vi "Read PSLabView Instance.vi"(8 "error in (no error)":errorcluster, 11 "PalmSens in":refnum<class "PalmSens.lvclass">) -> (0 "error out":errorcluster, 2 "PSLabView Instance":refnum<k24>, 3 "PalmSens out":refnum<class "PalmSens.lvclass">)   [LabVIEW 2025]
uses:
  PalmSens.lvclass/PalmSens.ctl
  PalmSens.lvclass
  C:/Users/stef/code/palmsenssdk/labview/PalmSens/Libraries/PalmSens.Core.Simplified.LabVIEW.dll
  Libraries/PalmSens.Core.Simplified.LabVIEW.dll
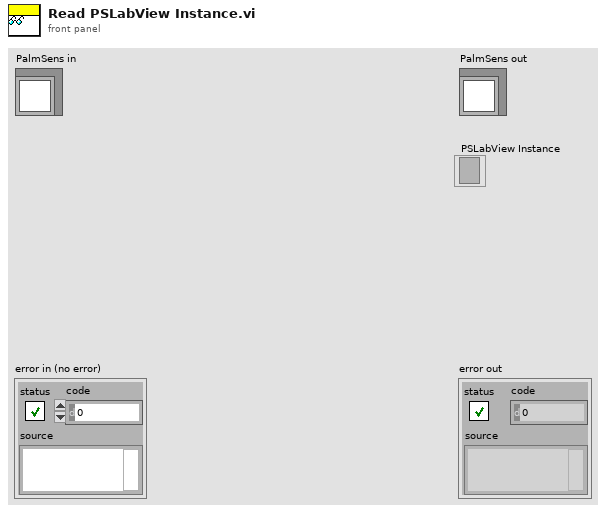
[diagram p1: front panel]
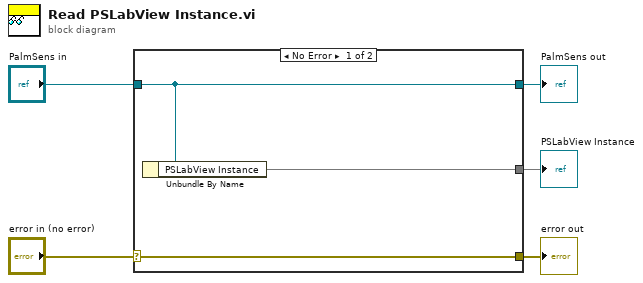
[diagram p0: block diagram]
diagram:
  n1 = case shown="No Error" "error in (no error)" {
    selector: "error in (no error)" -> [w8 w9]
    tunnel: [w8 w9] -> w4
    tunnel: [w7 w10] -> w2
    tunnel: "PalmSens in" -> [w7 w10]
    tunnel: [w6 _] -> w1
    frame No Error {
      n2 = Unbundle By Name(w7) -> ("PSLabView Instance"=w6)
    }
    frame Error {
    }
  }
  "error out" <- w4
  "PalmSens out" <- w2
  "PSLabView Instance" <- w1
